vi "Connect ICommunicate.vi"(8 "error in (no error)":errorcluster, 11 "CANopen Master in":refnum<class "CANopen Master.lvclass">) -> (0 "error out":errorcluster, 3 "CANopen Master out":refnum<class "CANopen Master.lvclass">)   [LabVIEW 2024, in "CANopen Master.lvclass"]
uses:
  CANopen Master/CANopen Master.lvclass
  CANopen Master/CANopen Master.lvclass/CANopen Master.ctl
  HAL/Source/Interfaces/IInitialize/IInitialize.lvclass
  HAL/Source/Interfaces/IRunnable/IRunnable.lvclass
  HAL/Source/Interfaces/IConfigurable/IConfigurable.lvclass
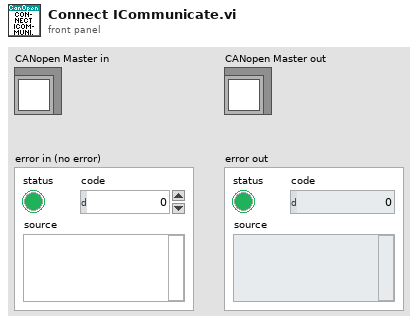
[diagram p1: front panel]
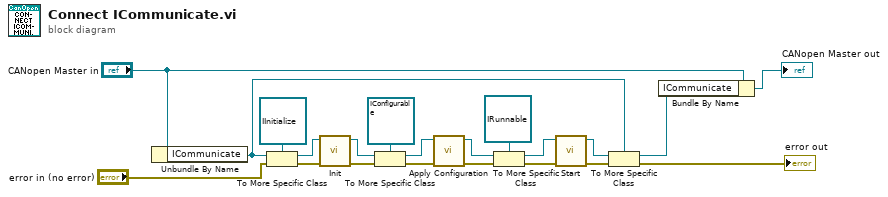
[diagram p0: block diagram]
diagram:
  n1 = Unbundle By Name("CANopen Master in") -> ("ICommunicate"=w9:refnum<class "ICommunicate.lvclass">)
  n2 = To More Specific Class(target class=refnum<class "IInitialize.lvclass"> refnum ("IInitialize.lvclass"), reference=w9, error in="error in (no error)") -> (specific class reference=w16:refnum<class "IInitialize.lvclass">, error out=w17:errorcluster)
  n3 = call-dynamic "Init.vi"("error in"=w17, "IInitialize in"=w16) -> ("error out"=w15:errorcluster, "IInitialize out"=w7:refnum<class "IInitialize.lvclass">)  [unwired: 8 in]
  n4 = To More Specific Class(target class=refnum<class "IConfigurable.lvclass"> refnum ("IConfigurable.lvclass"), reference=w7, error in=w15) -> (specific class reference=w4:refnum<class "IConfigurable.lvclass">, error out=w8:errorcluster)
  n5 = call-dynamic "Apply Configuration.vi"("error in"=w8, "IConfigurable in"=w4) -> ("error out"=w5:errorcluster, "IConfigurable out"=w3:refnum<class "IConfigurable.lvclass">)  [unwired: 8 in]
  n6 = To More Specific Class(target class=refnum<class "IRunnable.lvclass"> refnum ("IRunnable.lvclass"), reference=w3, error in=w5) -> (specific class reference=w11:refnum<class "IRunnable.lvclass">, error out=w14:errorcluster)
  n7 = call-dynamic "Start.vi"("error in"=w14, "IRunnable in"=w11) -> ("error out"=w12:errorcluster, "IRunnable out"=w10:refnum<class "IRunnable.lvclass">)  [unwired: 8 in]
  n8 = To More Specific Class(target class=w9, reference=w10, error in=w12) -> (specific class reference=w1:refnum<class "ICommunicate.lvclass">, error out=→"error out":errorcluster)
  n9 = Bundle By Name(cluster="CANopen Master in", "ICommunicate"=w1) -> (→"CANopen Master out":refnum<class "CANopen Master.lvclass">)
